vi "prototype UI.vi"() -> ()   [LabVIEW 2012]
uses:
  Custom Controls/Ch selector.ctl
  Custom Controls/MAIN Image panel tab Control type def.ctl
  Custom Controls/scan mode main settings tab.ctl
  Custom Controls/speed mode type def.ctl
  Custom Controls/pixel resolution enum.ctl
  Custom Controls/advanced settings inner tab CTL.ctl
  Custom Controls/Histogram tab.ctl
  Custom Controls/file format type def.ctl
  Custom Controls/experiment type.ctl
  Custom Controls/display palette control.ctl
  Custom Controls/PositionSaveMod.ctl
  <vilib>/event_ctls.llb/lveventtype.ctl
  GFG/GFG library.lvlib
panel:
  in  "PositionSaveButton":T1
  in  "reset zoom":bool
  out "Channel 5 large":T2(plugin-control)
  in  "bool.stage.speed":bool
  in  "Stage Stop":bool
  in  "step.size.xy":u16(ring)=6 items=["  1"=1, "  2"=2, "  5"=5, " 10"=10, " 20"=20, " 50"=50, "100"=100]
  in  "Y UP":bool
  in  "X LEFT":bool
  in  "Y DOWN":bool
  in  "X RIGHT":bool
  out "String 6":string
  in  "shutter":bool
  in  "x.pixels":i32=256 min=2 max=2048 step=2
  in  "clear prot":bool
  in  "timestamp.prot":bool
  in  "protocol.notes":string caption="notebook"
  in  "pos \nstore F":bool
  in  "pos \nstore E":bool
  in  "pos \nstore D":bool
  in  "pos \nstore C":bool
  in  "pos \nstore B":bool
  in  "pos \nstore A":bool
  out "String 10":string
  in  "pos \nrecall F":bool
  in  "pos \nrecall E":bool
  in  "pos \nrecall D":bool
  in  "pos \nrecall C":bool
  in  "pos \nrecall B":bool
  in  "pos \nrecall A":bool
  out "String 11":string
  in  "ref img\nOpen Files Button":bool
  in  "ref img\nstore F":bool
  in  "ref img\nstore E":bool
  in  "ref img\nstore D":bool
  in  "ref img\nstore C":bool
  in  "ref img\nstore B":bool
  in  "ref img\nstore A":bool
  out "String 17":string
  in  "ref img\nSave As Button":bool
  in  "Open All\nSettings":bool
  in  "step.size.z":u16(ring)=6 items=["  1"=1, "  2"=2, "  5"=5, " 10"=10, " 20"=20, " 50"=50, "100"=100]
  out "frame count":dbl(slide) scale=-1.0..280.0
  in  "scan mode main settings":T3
  in  "pixel resolution":T4
  in  "speed mode":T5=2 items=["extra fast scan", "fast scan", "standard scan", "long exposure"]
  in  "ROTATE":dbl(knob)=1.0 min=0.0 max=360.0 step=1.0 scale=0.0..360.0 scale format="%#_3g"
  in  "rotate.enable":bool
  in  "ZOOM":dbl(slide)=1.0 min=1.0 max=10.2 step=0.1 scale=1.0..8.0 scale format="%_2g"
  in  "no. of frames to acquire":i32=10000 min=2 max=2147483646 step=2
  in  "x.fov":dbl caption="Field of view    x" format="%#_3p"
  in  "y.fov":dbl caption="y" format="%#_3p"
  out "ms.p.line":dbl caption="ms/line" format="%#.2g"
  out "frames.p.sec":dbl caption="frames/s" format="%#.2g"
  out "pixels per line":i32=10000 min=2 max=2147483646 step=2
  out "lines per second":i32=10000 min=2 max=2147483646 step=2
  in  "linescan.y.pixels":i32=256 caption="Lines to display at once" min=2 max=2048 step=2
  in  "no. of lines to acquire":i32=10000 min=2 max=2147483646 step=2
  in  "experiment type":T6
  in  "experiment name":string
  in  "root.path":path=path "g:/"
  in  "Objective":u16(ring) items=["40x Olympus", "20x Olympus"]
  in  "file format":T7
  out "stack.duration":i32=10 caption="stack.duration (sec)" min=0 max=2147483646 step=2
  in  "add":bool
  in  "clear all":bool
  in  "clear last":bool
  in  "move to z.stack.\nstart plane":bool
  in  "start z.stack":bool
  in  "frames.per.plane":i32=10000
  in  "z.spacing":dbl=1.0 caption="z.spacing (um)" min=0.1 step=0.1
  out "no of planes":i32=10 min=0 max=2147483646 step=2
  in  "piezo.active":bool
  in  "frames.per.z.cycle":dbl=2.0 min=2.0 max=100.0 step=1.0
  in  "piezo.mode":bool
  in  "Z UP":bool
  in  "Z DOWN":bool
  out "String 7":string
  in  "setY":dbl caption="Z-Stepper" format="%#.1f"
  in  "setX":dbl caption="Z-Stepper" format="%#.1f"
  in  "setZ":dbl caption="set" format="%#.1f"
  out "String 4":string
  out "posZ":dbl caption="actual" format="%#.1f"
  out "posX":dbl caption="Z-Stepper" format="%#.1f"
  out "posY":dbl caption="Z-Stepper" format="%#.1f"
  out "String 3":string
  in  "XYZ stage settings slider tab":enum32{" "}(tab)
  in  "set stage speed":bool
  in  "enable virtual XYZ":bool
  out "String 16":string
  in  "set Y to zero":bool
  in  "set X to zero":bool
  in  "set all to zero":bool
  in  "set Z to zero":bool
  out "String 9":string
  in  "reverse y":bool
  in  "reverse x":bool
  in  "reverse z":bool
  out "String 8":string
  in  "PIN Button XYZ stage settings slider tab":bool
  in  "QUIT":bool
  in  "Record":bool
  in  "FOCUS":bool
  in  "MAIN Image panels":T8
  out "Channel 1 large":T2(plugin-control)
  out "Channel 2 large":T2(plugin-control)
  out "Channel 3 large":T2(plugin-control)
  out "Channel 4 large":T2(plugin-control)
  out "Channel 1 small":T2(plugin-control)
  out "Channel 2 small":T2(plugin-control)
  out "Channel 4 small":T2(plugin-control)
  out "Channel 3 small":T2(plugin-control)
  in  "Blue Channel (Overlay)":T9 caption="B"
  in  "Green Channel (Overlay)":T9=enum."Ch 1" caption="G"
  in  "Red Channel (Overlay)":T9=enum."Ch 2" caption="R"
  out "RGB overlay":T2(plugin-control)
  out "ROI chart":sgl[][](graph)=[[54.570076, 54.556858]]
  in  "ROI channel":T9=enum."Ch 1" caption="Channel"
  out "ROI Image display":T2(plugin-control)
  in  "load coordinates":bool
  in  "confirm line":bool
  in  "channel arb line scan":T9 caption="Channel"
  out "arb line scan display":T2(plugin-control)
  in  "Cancel":bool
  in  "hist/ref slider tab":enum32{" "}(tab)
  in  "PIN Button hist/ref slider tab":bool
  in  "Histograms tab":T10
  in  "auto scale\n      CH 1":bool=TRUE caption="auto scale 2"
  in  "Min Max Channel 1":cluster{dbl, dbl}(slide) scale=-100.0..2047.0 scale format="%#_4g"
  out "Histogram 1":T11(graph)
  out "String 12":string
  in  "auto scale\n      CH 4":bool=TRUE caption="auto scale 2"
  in  "Min Max Channel 4":cluster{dbl, dbl}(slide) scale=-100.0..2047.0 scale format="%#_4g"
  out "Histogram 4":T11(graph)
  out "String 15":string
  in  "auto scale\n      CH 3":bool=TRUE caption="auto scale 2"
  in  "Min Max Channel 3":cluster{dbl, dbl}(slide) scale=-100.0..2047.0 scale format="%#_4g"
  out "Histogram 3":T11(graph)
  out "String 14":string
  in  "auto scale\n      CH 2":bool=TRUE caption="auto scale 2"
  in  "Min Max Channel 2":cluster{dbl, dbl}(slide) scale=-100.0..2047.0 scale format="%#_4g"
  out "Histogram 2":T11(graph)
  out "String 13":string
  in  "avg type":u16(ring) items=["none", "group avg", "moving avg"]
  in  "avg of":i8=10 min=2 step=1
  in  "display palette":T12
  in  "laser power slider tab":enum32{""}(tab)
  in  "enable set power max":bool
  in  "set power max":bool
  in  "Laser Power":dbl(knob) step=0.5 scale=0.0..100.0 scale format="%3d"
  in  "PIN Button laser power slider tab":bool
  in  "PMT slider tab":enum32{""}(tab)
  in  "PMT 2":u16(slide) max=1000 scale=0.0..1000.0
  in  "PMT 1":u16(slide) max=1250 scale=0.0..1000.0
  out "String 5":string
  in  "PMT 4":u16(slide) max=1000 scale=0.0..1000.0
  in  "PMT 3":u16(slide) max=1250 scale=0.0..1000.0
  out "String 18":string
  in  "PIN Button PMT slider tab":bool
  in  "advanced settings slider tab":enum32{""}(tab)
  in  "advanced settings inner tab":T13
  in  "pixel.dwell.time.in.sec":dbl=1e-05 min=4e-07 max=1e-05 step=2e-07 format="%#.6p"
  in  "y.pixel.sz":dbl=1e-05 min=1e-09 max=1e-05 step=1e-07 format="%#_3p"
  in  "x.pixel.sz":dbl=1e-05 min=1e-09 max=1e-05 step=1e-07 format="%#_3p"
  in  "y.pixels":i32=256 caption="Y Resolution" min=2 max=2048 step=2
  in  "fill fraction":dbl=60.0 caption="%" min=60.0 max=100.0 step=0.5 format="%_3g"
  in  "nomin.x.pixels":i32=256 caption="X resolution" min=2 max=2048 step=2
  in  "y bidirectional":bool
  in  "x bidirectional":bool=TRUE
  in  "max.field.of.view":dbl=300.0 format="%#_6p"
  in  "voltage.for\nmax.field.of.view":dbl=5.0
  in  "x.voltage":dbl=0.9999999999999999 min=0.0 max=5.5 step=0.1
  in  "y.voltage":dbl=1.0 min=0.0 max=5.5 step=0.1
  in  "y.volt.offset":dbl=-0.2 step=0.1
  in  "x.volt.offset":dbl=-0.2 step=0.1
  in  "pixel.dwell.time.in.ticks":u16=20 min=2 step=1
  in  "sample.clock":dbl=5000000.0
  in  "Start.Delay":dbl=100.0 min=1.0 step=1.0
  out "ADsamples.per.frame":i32
  in  "ai.active3":bool
  in  "ai.active2":bool
  in  "ai.active1":bool
  in  "ai.active0":bool caption="active?"
  in  "ai.range2":dbl=10.0 min=0.1 max=10.0 step=0.1
  in  "ai.range1":dbl=10.0 min=0.1 max=10.0 step=0.1
  out "ai.string3":string
  out "ai.string2":string
  out "ai.string1":string
  out "ai.string0":string caption="Analog Input"
  in  "ai.range0":dbl=10.0 caption="input range" min=0.1 max=10.0 step=0.1
  in  "ai.range3":dbl=10.0 min=0.1 max=10.0 step=0.1
  in  "external.start.trigger.enable":bool=TRUE caption="WAIT FOR TRIGGER"
  in  "pos  pockels cell PMT Data":dbl[][](array[numeric])=[[0.0, 0.0], [1.0, 0.0]] caption="Data" format="%0.1f"
  out "interpol XY":cluster{dbl[], "Best Exponential Fit":dbl[]}[](graph)
  in  "PIN Button advanced settings slider tab":bool
  in  "SCIENTIFICA Button":bool
  # "to zoom out press and hold Shift"
  # "current pos."
  # "go to pos."
  # "STORE positions"
  # "RECALL  positions"
  # "REFERENCE IMAGES"
  # "STORE"
  # "zig-zag (leaf scan)"
  # "planes"
  # "virtual XYZ"
  # "set zero"
  # "reverse \ndirection"
  # "1"
  # "2"
  # "3"
  # "4"
  # "Press and hold Ctrl to add multriple ROIs"
  # "This checkbox is only for starting the image acquisition using a TTL rising edge trigger from an external device. Don't tick this box unless an incoming trigger is wired up, otherwise the software may freeze. To reset, click QUIT and restart. If you want to send a trigger to an external device, just connect the ai.start.trigger.channel (e.g.PFI2, specified in settings.INI) to the external device, but leave the  checkbox above unticked."
  # "Z"
  # "laser"
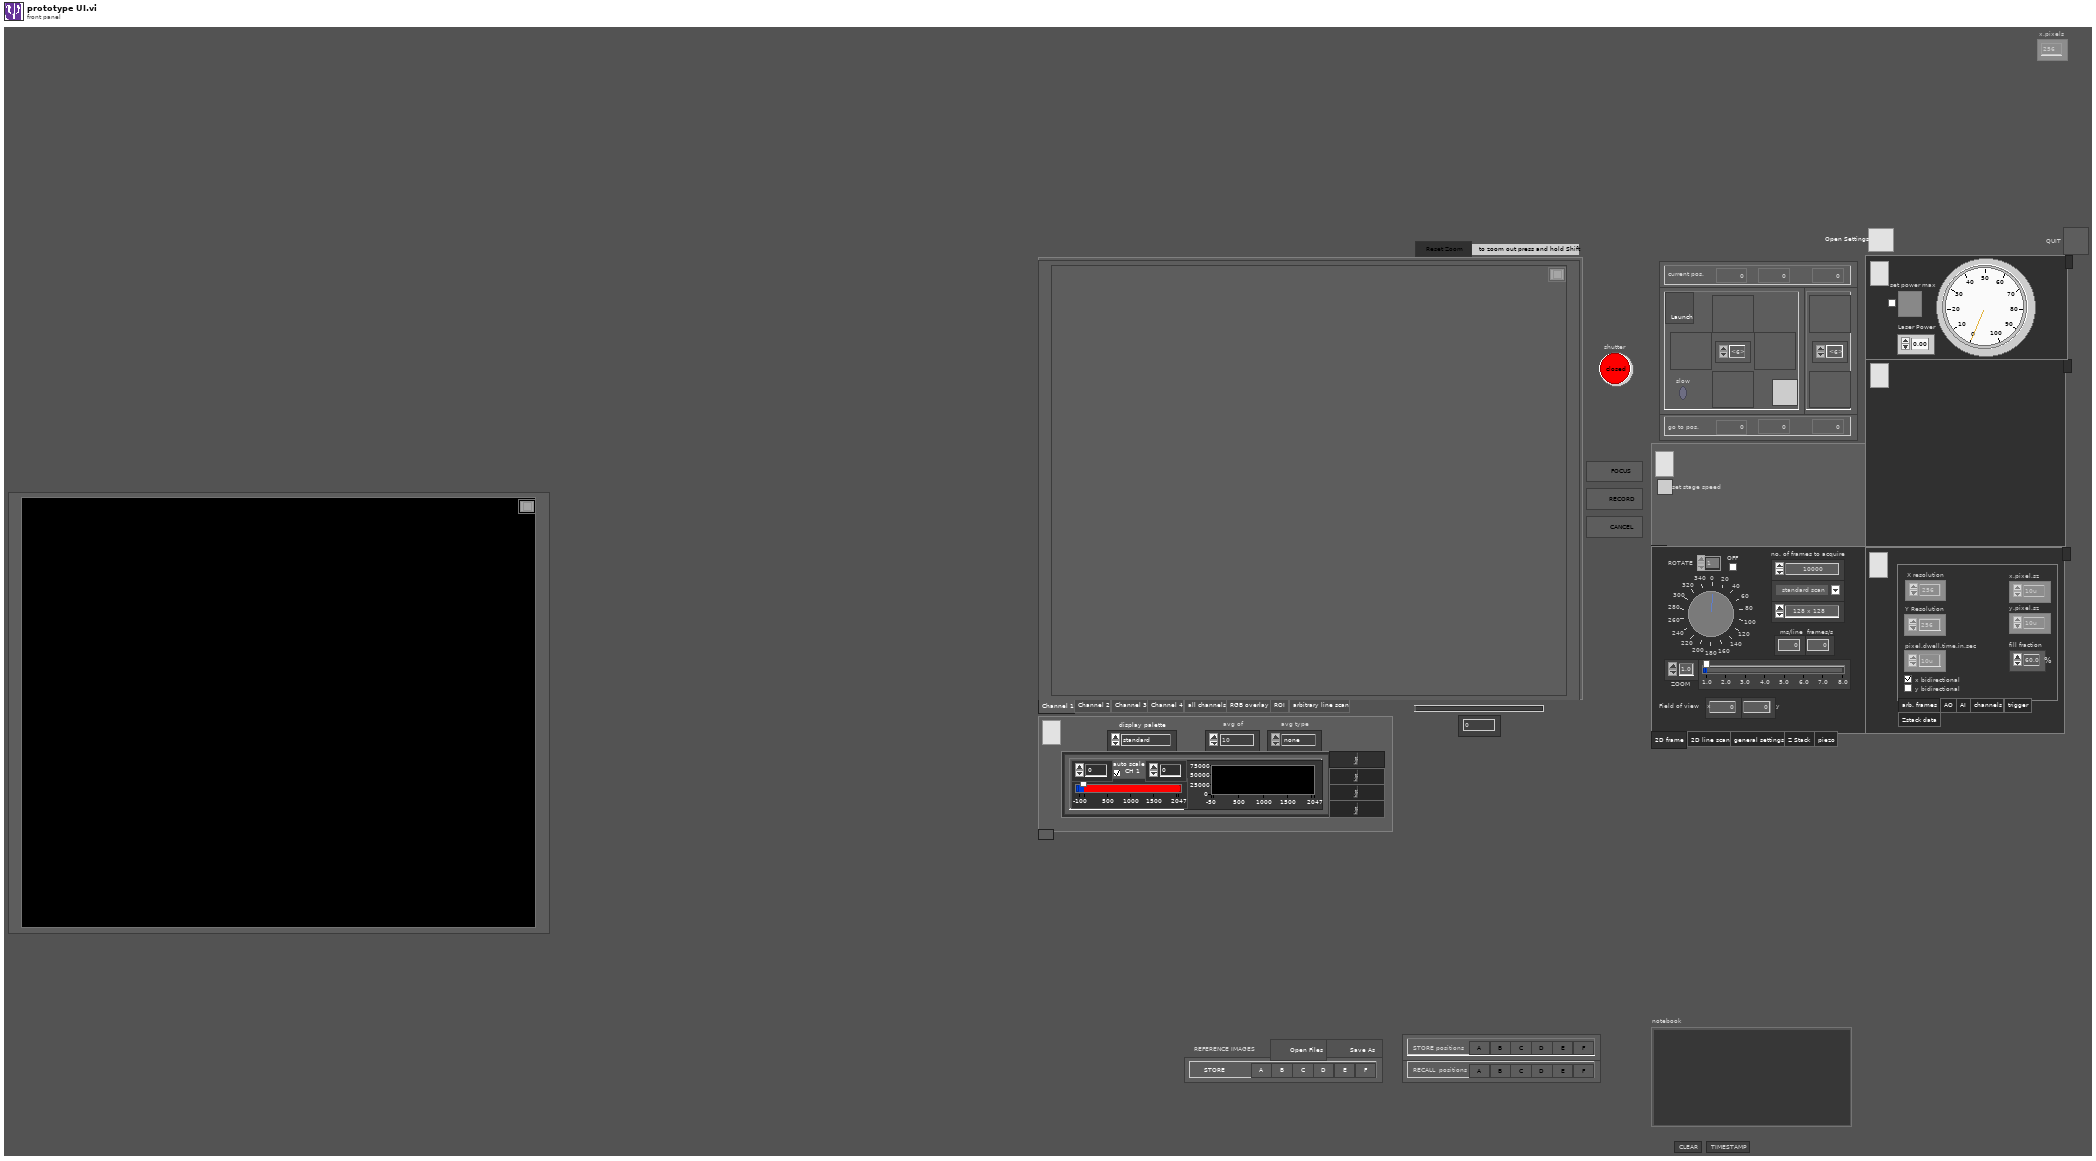
[diagram p1: front panel]
types:
  T1 = typedef "PositionSaveMod.ctl" = bool
  T2 = typedef "IMAQ Image.ctl" = refnum<image>
  T3 = typedef "scan mode main settings tab.ctl" = enum32{"2D frame", "2D line scan", "general settings", "Z Stack", "piezo"}
  T4 = typedef "pixel resolution enum.ctl" = enum16{"   128 x 128", "   256 x 128", "   256 x 256", "   512 x  64", "   512 x 128", "   512 x 256", "   512 x 512", "  1024 x 512", "  1024 x 1024", "   arbitrary"}
  T5 = typedef "speed mode type def.ctl" = u16
  T6 = typedef "experiment type.ctl" = string
  T7 = typedef "file format type def.ctl" = enum16{"16bit raw", "32bit raw", "16bit multi-tiff (interleave)", "16bit multi-tiff (separate)", "16bit multi-tiff (stacked)", "32bit multi-tiff (interleave)", "32bit multi-tiff (separate)", "32bit multi-tiff (stacked)", "16bit tiff series (interleave)", "16bit tiff series (separate)", "16bit tiff series (stacked)", "32bit tiff series (interleave)", "32bit tiff series (separate)", "32bit tiff series (stacked)"}
  T8 = typedef "MAIN Image panel tab Control type def.ctl" = enum32{"Channel 1", "Channel 2", "Channel 3", "Channel 4", "all channels", "RGB overlay", "ROI", "arbitrary line scan"}
  T9 = typedef "Ch selector.ctl" = enum16{"none", "Ch 1", "Ch 2", "Ch 3", "Ch 4", "Ch 5"}
  T10 = typedef "Histogram tab.ctl" = enum32{"hist Ch 1", "hist Ch 4", "hist Ch 3", "hist Ch 2"}
  T11 = cluster{"Starting Value":sgl, "Incremental Value":sgl, "Histogram":u32[]}
  T12 = typedef "display palette control.ctl" = enum16{"standard", "high clipping red", "low clipping blue", "high and low clipping"}
  T13 = typedef "advanced settings inner tab CTL.ctl" = enum32{"arb. frames", "AO", "AI", "channels", "trigger", "Zstack data"}
  T14 = enum8{"Enabled", "Disabled", "Disabled and Grayed Out"}
  T15 = typedef "Image Type" = u32
  T16 = cluster{refnum<vi>, refnum<vi>, refnum<vi>, refnum<vi>, refnum<vi>, refnum<vi>, refnum<vi>, refnum<vi>, refnum<vi>, refnum<vi>, refnum<vi>, refnum<vi>}
  T17 = cluster{"New Image":T2, "New Image":T2, "New Image":T2, "New Image":T2, "New Image":T2, "New Image":T2, "New Image":T2, "New Image":T2, "New Image":T2, "New Image":T2, "New Image":T2, "New Image":T2}
  T18 = typedef "lveventtype.ctl" = enum32{"Null", "Timeout", "Annotation Menu Selection", "Annotation Menu Selection?", "App Instance Close", "App Instance Close?", "Autoscale Range Change", "Cell Edit", "Cell Edit?", "Cursor Grab", "Cursor Grab?", "Cursor Menu Selection", "Cursor Menu Selection?", "Cursor Move", "Cursor Release", "Data Change", "Direction Change", "Display State Change", "Drag Ended", "Drag Enter", "Drag Leave", "Drag Over", "Drag Source Update", "Drag Starting", "Drag Starting?", "Drop", "Exec State Change", "Key Down", "Key Down?", "Key Repeat", "Key Repeat?", "Key Up", "Listbox Double Click", "Menu Activation?", "Menu Selection (App)", "Menu Selection? (App)", "Menu Selection (User)", "Mouse Down", "Mouse Down?", "Mouse Enter", "Mouse Leave", "Mouse Move", "Mouse Up", "NI Security User Change (App)", "Pane Size", "Panel Close", "Panel Close?", "Panel Resize", "Plot Attribute Change", "Scale Range Change", "Shortcut Menu Activation?", "Shortcut Menu Selection (App)", "Shortcut Menu Selection? (App)", "Shortcut Menu Selection (User)", "Tree Double Click", "Tree Drag", "Tree Drag?", "Tree Drop", "Tree Drop?", "Tree Item Close", "Tree Item Close?", "Tree Item Open", "Tree Item Open?", "Value Change"}
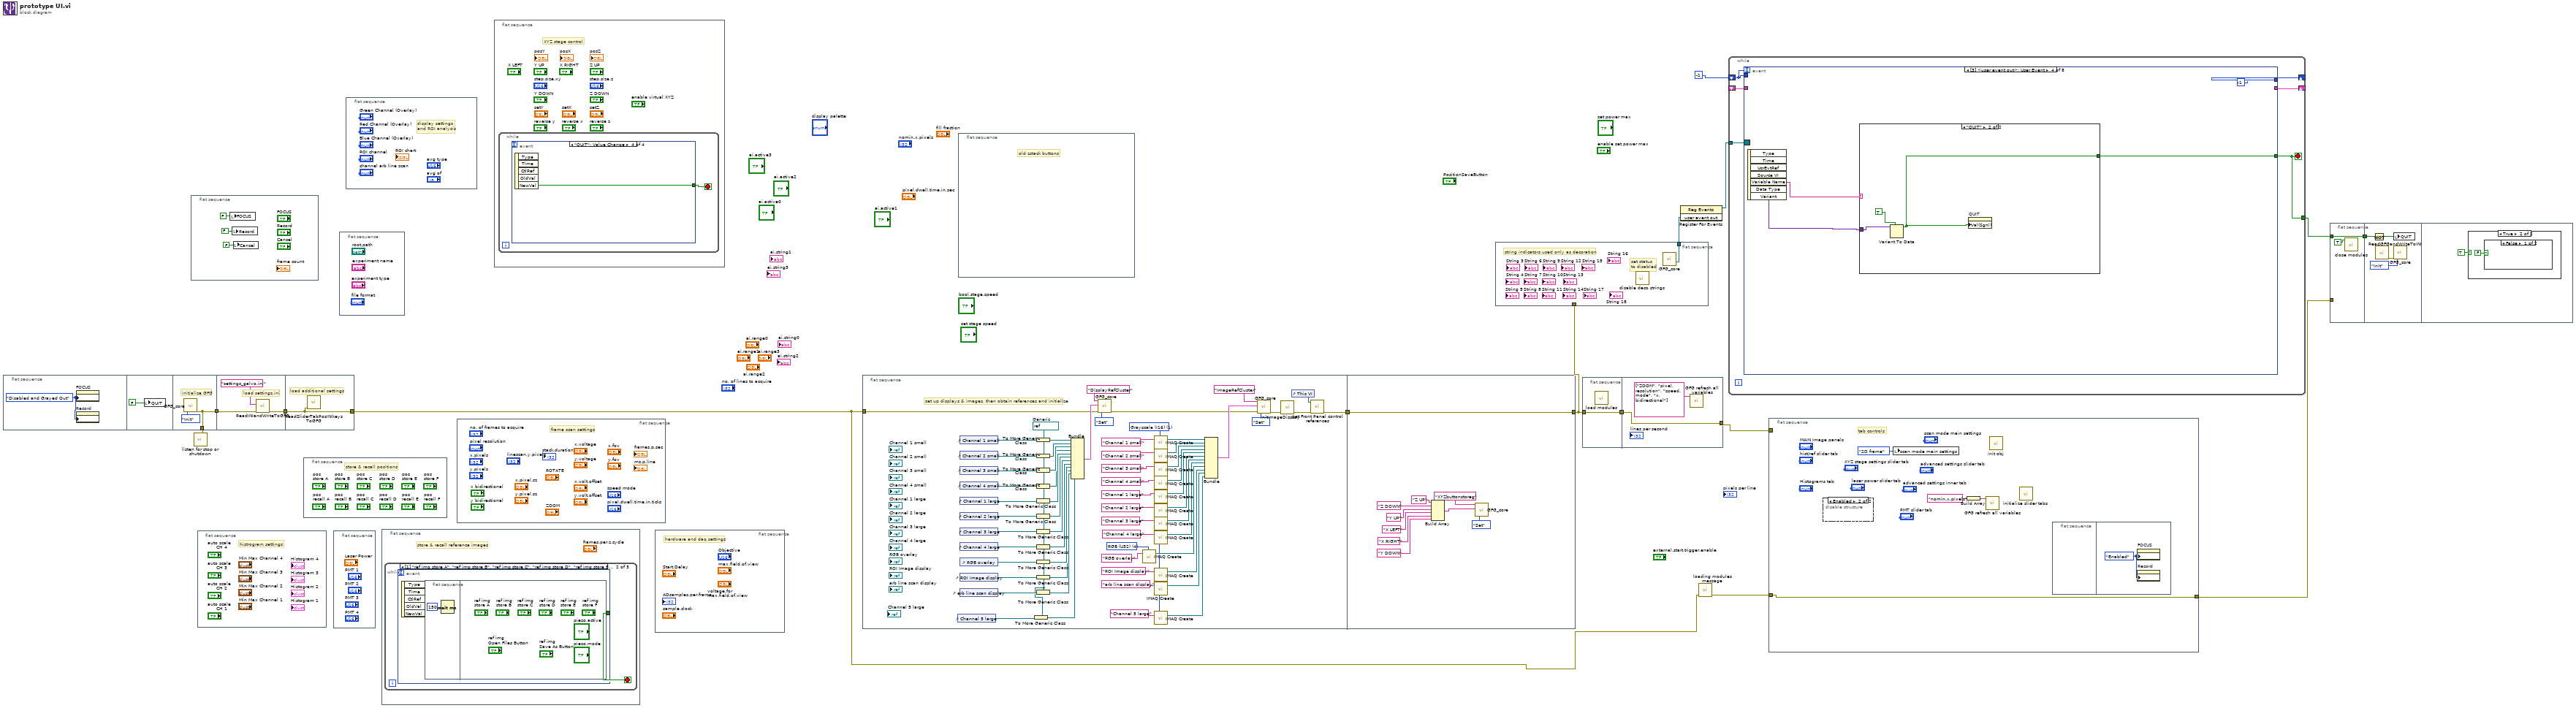
[diagram p0: block diagram]
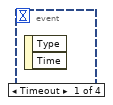
[diagram p2: hidden frame]
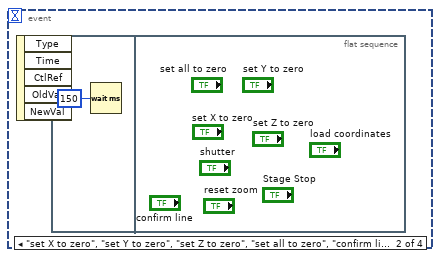
[diagram p3: hidden frame]
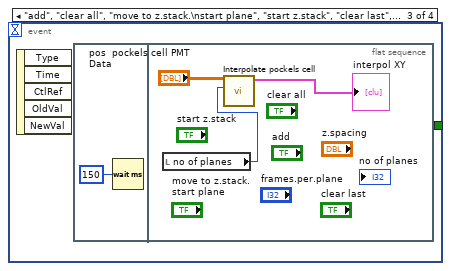
[diagram p4: hidden frame]
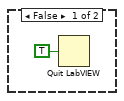
[diagram p5: hidden frame]
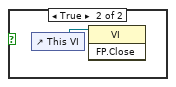
[diagram p6: hidden frame]
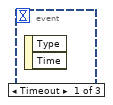
[diagram p7: hidden frame]
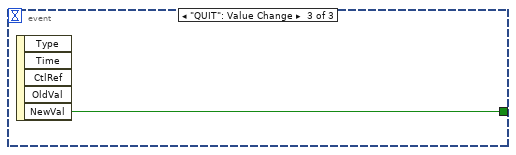
[diagram p8: hidden frame]
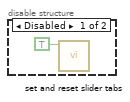
[diagram p9: hidden frame]
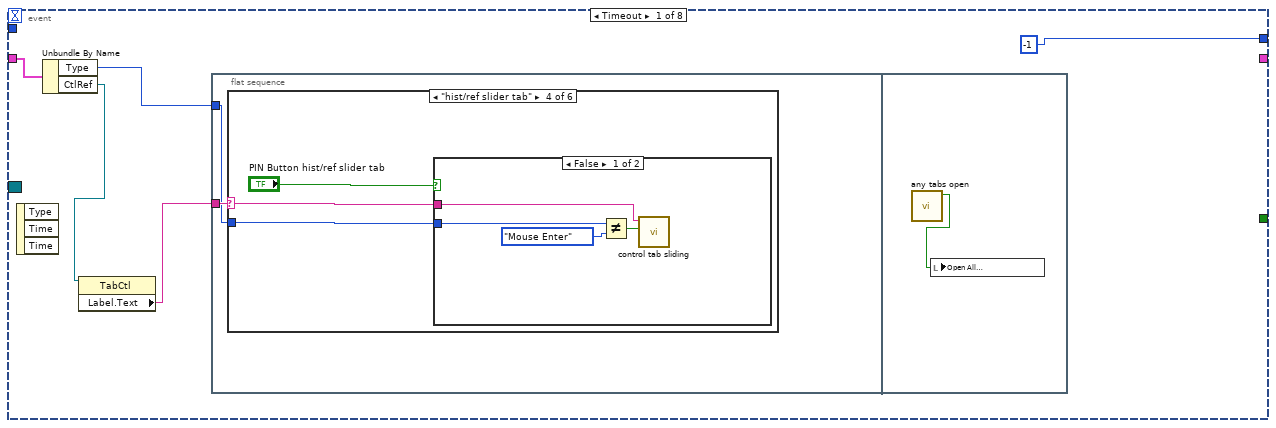
[diagram p10: hidden frame]
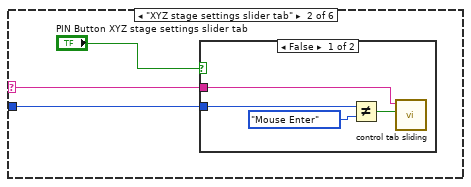
[diagram p12: hidden frame]
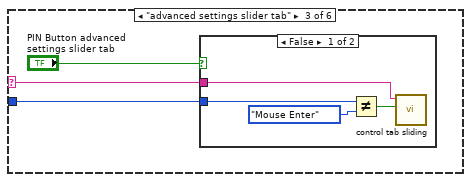
[diagram p14: hidden frame]
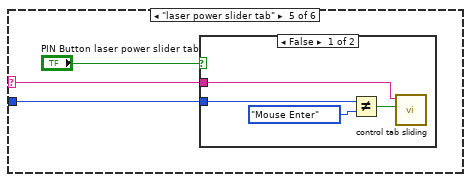
[diagram p17: hidden frame]
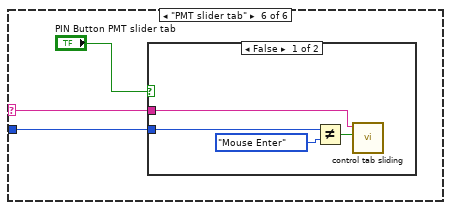
[diagram p19: hidden frame]
diagram:
  n1 = flat-sequence {
    tunnel: [w18] -> w15
    tunnel: [w18] -> w14
    tunnel: w15 -> [w22]
    tunnel: [w21] -> w9
    tunnel: [w23] -> w4
    tunnel: w9 -> [w23]
    frame #0 {
      w16 = T14."Disabled and Grayed Out" ("Disabled")
      n2 = property on="FOCUS" class="Bool (strict)"("DisabledEnum"=w16) -> ()  [unwired: 2 in, 2 out]
      n3 = property on="Record" class="Bool (strict)"("DisabledEnum"=w16) -> ()  [unwired: 2 in, 2 out]
    }
    frame #1 {
      n4 = local write "QUIT"(FALSE ("QUIT")) -> ()
    }
    frame #2 {
      # "initialize GFG"
      n5 = call "GFG_core.vi"("Action"=enum16{"Init", "Set", "Get"}."Init") -> ("error out"=w18:errorcluster)  [unwired: 12 in, 6 out]
    }
    frame #3 {
      # "load settings.ini"
      n6 = call "ReadINIandWriteToGFG.vi"("error in (no error)"=w22, "name or relative path"="settings_galvo.ini") -> ("error out"=w21:errorcluster)  [unwired: 9 in]
    }
    frame #4 {
      # "load additional settings"
      n7 = call "ReadSliderTabPosINIkeysToGFG.vi"("error in (no error)"=w23) -> ()  [unwired: 11 in]
    }
  }
  n8 = flat-sequence {
    frame #0 {
      n9 = local write "FOCUS"(FALSE ("FOCUS")) -> ()
      n10 = local write "Record"(FALSE ("Record")) -> ()
      n11 = local write "Cancel"(FALSE ("Cancel")) -> ()
    }
  }
  n12 = call "listen for stop or shutdown.vi"("error in (no error)"=w14) -> ()  [unwired: 9 in, 2 out]
  n13 = flat-sequence {
    frame #0 {
      # "histrogram settings"
    }
  }
  n14 = flat-sequence {
    frame #0 {
      # "store & recall positions"
    }
  }
  n15 = flat-sequence {
    frame #0 {
    }
  }
  n16 = flat-sequence {
    frame #0 {
    }
  }
  n17 = flat-sequence {
    frame #0 {
      # "display settings\nand ROI analysis"
    }
  }
  n18 = flat-sequence {
    frame #0 {
      # "store & recall reference images"
      n19 = while {
        stop <- w27 stop-if-true
        n20 = event shown="[1] \"ref img store A\", \"ref img store B\", \"ref img store C\", \"ref img store D\", \"ref img store E\", \"ref img store F\", \"ref img Save As Button\", \"ref img Open Files Button\": Value Change" {
          selector: _ -> [_ _ _]
          dyn-events: _ -> [_ _ _]
          timeout: _ -> [_ _ _]
          tunnel: [_ _ w29] -> w27
          event Timeout {
            n21 = event-data() -> ()  [unwired: 1 in, 2 out]
          }
          event "ref img\nstore A", "ref img\nstore B", "ref img\nstore C", "ref img\nstore D", "ref img\nstore E", "ref img\nstore F", "ref img\nSave As Button", "ref img\nOpen Files Button": Value Change {
            n22 = event-data() -> ()  [unwired: 1 in, 5 out]
            n23 = flat-sequence {
              frame #0 {
                n24 = Wait (ms)(milliseconds to wait=u32 150) -> ()  [unwired: 1 out]
              }
              frame #1 {
              }
            }
          }
          event "QUIT": Value Change {
            n25 = event-data() -> ("NewVal"=w29:bool)  [unwired: 1 in, 4 out]
          }
        }
      }
    }
  }
  n26 = flat-sequence {
    frame #0 {
      # "frame scan settings"
    }
  }
  n27 = flat-sequence {
    frame #0 {
      # "XYZ stage control"
      n28 = while {
        stop <- w30 stop-if-true
        n29 = event shown="[3] \"QUIT\": Value Change" {
          selector: _ -> [_ _ _ _]
          dyn-events: _ -> [_ _ _ _]
          timeout: _ -> [_ _ _ _]
          tunnel: [_ _ _ w36] -> w30
          event Timeout {
            n30 = event-data() -> ()  [unwired: 1 in, 2 out]
          }
          event "set X to zero", "set Y to zero", "set Z to zero", "set all to zero", "confirm line", "Stage Stop", "reset zoom": Value Change {
            n31 = event-data() -> ()  [unwired: 1 in, 5 out]
            n32 = flat-sequence {
              frame #0 {
                n33 = Wait (ms)(milliseconds to wait=u32 150) -> ()  [unwired: 1 out]
              }
              frame #1 {
              }
            }
          }
          event "add", "clear all", "move to z.stack.\nstart plane", "start z.stack", "clear last", "z.spacing", "frames.per.plane", "no of planes", "pos  pockels cell PMT Data": Value Change {
            n34 = event-data() -> ()  [unwired: 1 in, 5 out]
            n35 = flat-sequence {
              frame #0 {
                n36 = Wait (ms)(milliseconds to wait=u32 150) -> ()  [unwired: 1 out]
              }
              frame #1 {
                n37 = local read "no of planes"() -> (w33:i32)
                n38 = call "Interpolate pockels cell.vi"("nr of planes"=w33, "Data"="pos  pockels cell PMT Data") -> ("Raw Data and Interpolated Data"=→"interpol XY":cluster{dbl[], "Best Exponential Fit":dbl[]}[])  [unwired: 8 in, 1 out]
              }
            }
          }
          event "QUIT": Value Change {
            n39 = event-data() -> ("NewVal"=w36:bool)  [unwired: 1 in, 4 out]
          }
        }
      }
    }
  }
  n40 = flat-sequence {
    frame #0 {
      # "hardware and daq settings"
    }
  }
  n41 = flat-sequence {
    tunnel: w4 -> [w56]
    tunnel: [w37] -> w6
    tunnel: [w109] -> w12
    tunnel: w6 -> [w109]
    frame #0 {
      w44 = T15 4 items=["Grayscale (U8)", "Grayscale (I16)", "Grayscale (SGL)", "Complex (CSG)", "RGB (U32)", "HSL (U32)", "RGB (U64)", "Grayscale (U16)"] ("Image Type")
      w39 = T15 1 items=["Grayscale (U8)", "Grayscale (I16)", "Grayscale (SGL)", "Complex (CSG)", "RGB (U32)", "HSL (U32)", "RGB (U64)", "Grayscale (U16)"] ("Image Type")
      w41 = refnum<vi> refnum  # Generic
      # "set up displays & images, then obtain references and initialize"
      n42 = control-ref of="Channel 5 large"() -> (w43:refnum<vi>)
      n43 = control-ref of="Channel 1 small"() -> (w55:refnum<vi>)
      n44 = control-ref of="Channel 2 small"() -> (w54:refnum<vi>)
      n45 = control-ref of="Channel 3 small"() -> (w53:refnum<vi>)
      n46 = control-ref of="Channel 4 small"() -> (w52:refnum<vi>)
      n47 = control-ref of="Channel 1 large"() -> (w51:refnum<vi>)
      n48 = control-ref of="Channel 2 large"() -> (w50:refnum<vi>)
      n49 = control-ref of="Channel 3 large"() -> (w49:refnum<vi>)
      n50 = control-ref of="Channel 4 large"() -> (w48:refnum<vi>)
      n51 = control-ref of="RGB overlay"() -> (w47:refnum<vi>)
      n52 = control-ref of="ROI Image display"() -> (w46:refnum<vi>)
      n53 = control-ref of="arb line scan display"() -> (w45:refnum<vi>)
      n54 = To More Generic Class(target class=w41, reference=w43) -> (generic class reference=w40:refnum<vi>)
      n55 = To More Generic Class(target class=w41, reference=w55) -> (generic class reference=w96:refnum<vi>)
      n56 = To More Generic Class(target class=w41, reference=w54) -> (generic class reference=w89:refnum<vi>)
      n57 = To More Generic Class(target class=w41, reference=w53) -> (generic class reference=w88:refnum<vi>)
      n58 = To More Generic Class(target class=w41, reference=w52) -> (generic class reference=w87:refnum<vi>)
      n59 = To More Generic Class(target class=w41, reference=w51) -> (generic class reference=w86:refnum<vi>)
      n60 = To More Generic Class(target class=w41, reference=w50) -> (generic class reference=w95:refnum<vi>)
      n61 = To More Generic Class(target class=w41, reference=w49) -> (generic class reference=w94:refnum<vi>)
      n62 = To More Generic Class(target class=w41, reference=w48) -> (generic class reference=w93:refnum<vi>)
      n63 = To More Generic Class(target class=w41, reference=w47) -> (generic class reference=w92:refnum<vi>)
      n64 = To More Generic Class(target class=w41, reference=w46) -> (generic class reference=w91:refnum<vi>)
      n65 = To More Generic Class(target class=w41, reference=w45) -> (generic class reference=w90:refnum<vi>)
      n66 = Bundle(w96, w89, w88, w87, w86, w95, w94, w93, w92, w91, w90, w40) -> (w99:T16)  [unwired: 1 in]
      n67 = call "GFG_core.vi"("Variable Name in"="DisplayRefCluster", "Variant in"=w99, "error in (no error)"=w56, "Action"=enum16{"Init", "Set", "Get"}."Set") -> ("error out"=w60:errorcluster)  [unwired: 9 in, 6 out]
      n68 = call "IMAQ Create"("Image Name"="RGB overlay", "Image Type"=w44) -> ("New Image"=w80:T2)  [unwired: 3 in, 1 out]
      n69 = call "IMAQ Create"("Image Name"="Channel 1 small", "Image Type"=w39) -> ("New Image"=w72:T2)  [unwired: 3 in, 1 out]
      n70 = call "IMAQ Create"("Image Name"="Channel 2 small", "Image Type"=w39) -> ("New Image"=w73:T2)  [unwired: 3 in, 1 out]
      n71 = call "IMAQ Create"("Image Name"="Channel 3 small", "Image Type"=w39) -> ("New Image"=w74:T2)  [unwired: 3 in, 1 out]
      n72 = call "IMAQ Create"("Image Name"="Channel 4 small", "Image Type"=w39) -> ("New Image"=w75:T2)  [unwired: 3 in, 1 out]
      n73 = call "IMAQ Create"("Image Name"="Channel 1 large", "Image Type"=w39) -> ("New Image"=w76:T2)  [unwired: 3 in, 1 out]
      n74 = call "IMAQ Create"("Image Name"="Channel 2 large", "Image Type"=w39) -> ("New Image"=w77:T2)  [unwired: 3 in, 1 out]
      n75 = call "IMAQ Create"("Image Name"="Channel 3 large", "Image Type"=w39) -> ("New Image"=w78:T2)  [unwired: 3 in, 1 out]
      n76 = call "IMAQ Create"("Image Name"="Channel 4 large", "Image Type"=w39) -> ("New Image"=w79:T2)  [unwired: 3 in, 1 out]
      n77 = call "IMAQ Create"("Image Name"="ROI Image display", "Image Type"=w39) -> ("New Image"=w81:T2)  [unwired: 3 in, 1 out]
      n78 = call "IMAQ Create"("Image Name"="arb line scan display", "Image Type"=w39) -> ("New Image"=w82:T2)  [unwired: 3 in, 1 out]
      n79 = call "IMAQ Create"("Image Name"="Channel 5 large", "Image Type"=w39) -> ("New Image"=w38:T2)  [unwired: 3 in, 1 out]
      n80 = Bundle("New Image"=w72, "New Image"=w73, "New Image"=w74, "New Image"=w75, "New Image"=w76, "New Image"=w77, "New Image"=w78, "New Image"=w79, "New Image"=w80, "New Image"=w81, "New Image"=w82, "New Image"=w38) -> (w84:T17)  [unwired: 1 in]
      n81 = call "GFG_core.vi"("Variable Name in"="ImageRefCluster", "Variant in"=w84, "error in (no error)"=w60, "Action"=enum16{"Init", "Set", "Get"}."Set") -> ("error out"=w59:errorcluster)  [unwired: 9 in, 6 out]
      n82 = call "InitImageDisplay.vi"("error in (no error)"=w59) -> ("error out"=w58:errorcluster)  [unwired: 10 in]
      n83 = control-ref of="This VI"() -> (w57:refnum<vi>)
      n84 = call "get Front Panel control references.vi"("error in (no error)"=w58, "Main VI"=w57) -> ("error out"=w37:errorcluster)  [unwired: 9 in]
    }
    frame #1 {
      n85 = Build Array("Z UP" ("Variable Name in"), "Z DOWN" ("Variable Name in"), "Y UP" ("Variable Name in"), "X LEFT" ("Variable Name in"), "X RIGHT" ("Variable Name in"), "Y DOWN" ("Variable Name in")) -> (w100:string[])
      n86 = call "GFG_core.vi"("Variable Name in"="XYZbuttonstoreg", "Variant in"=w100, "Action"=enum16{"Init", "Set", "Get"}."Set") -> ()  [unwired: 10 in, 7 out]
    }
  }
  n87 = flat-sequence {
    frame #0 {
      # "old zstack buttons"
    }
  }
  n88 = flat-sequence {
    tunnel: w12 -> [_]
    tunnel: [w110] -> w2
    frame #0 {
      # "set status\nto disabled"
      # "string indicators used only as decoration"
      n89 = call "disable deco strings.vi"() -> ()  [unwired: 11 in, 1 out]
      n90 = call "GFG_core.vi"() -> ("user event out"=w110:refnum<user-event>)  [unwired: 13 in, 6 out]
    }
  }
  n91 = flat-sequence {
    tunnel: w12 -> [w111]
    tunnel: [w111] -> w8
    tunnel: [w113] -> w7
    tunnel: w8 -> [w113]
    frame #0 {
      n92 = call "load modules.vi"() -> ()  [unwired: 12 in]
    }
    frame #1 {
      n93 = call "GFG refresh all variables.vi"("Variables to refresh"=string[] ["ZOOM", "pixel.resolution", "speed.mode", "x.bidirectional"] ("Variables Names In")) -> ()  [unwired: 11 in]
    }
  }
  n94 = register-events(w2) -> (reference out=w3:refnum<event-registration>)  [unwired: 2 in, 1 out]
  n95 = call "loading modules message.vi"("error in"=w4) -> ("error out"=w5:errorcluster)  [unwired: 10 in]
  n96 = while {
    tunnel: [w119] -> w13
    shift-right: [w118] -> _
    shift-left: _ -> [w116]
    shift-right: [w117] -> _
    shift-left: -1 -> [w115]
    tunnel: w3 -> [w114]
    stop <- w119 stop-if-true
    n97 = event shown="[3] <user event out>: User Event" {
      selector: w114 -> [_ _ _ _ _ _ _ _]
      dyn-events: _ -> [_ _ _ _ _ _ _ _]
      timeout: w115 -> [_ _ _ _ _ _ _ _]
      tunnel: [_ _ "QUIT" w177 _ _ _ _] -> w119
      tunnel: [_ _ _ _ _ _ w191 _] -> w118
      tunnel: [-1 w163 w174 -1 w183 w185 w195 w205] -> w117
      tunnel: w116 -> [w124 _ _ _ _ _ w190 _]
      tunnel: w115 -> [_ w163 w174 _ w183 w185 w194 w205]
      event Timeout {
        n98 = event-data() -> ()  [unwired: 1 in, 3 out]
        n99 = Unbundle By Name(w124) -> ("Type"=w121:T18, "CtlRef"=w123:refnum<vi>)
        n100 = property class="TabCtl"(reference=w123) -> ("Label.Text"=w122:string)  [unwired: 1 in, 2 out]
        n101 = flat-sequence {
          tunnel: w122 -> [w126]
          tunnel: w121 -> [w125]
          frame #0 {
            n102 = case shown="\"hist/ref slider tab\"" w126 {
              selector: w126 -> [_ w128 w134 w143 w148 w157]
              tunnel: w125 -> [_ w127 w135 w141 w149 w156]
              frame "False", Default {
              }
              frame "XYZ stage settings slider tab" {
                n103 = case shown="False" "PIN Button XYZ stage settings slider tab" {
                  tunnel: w128 -> [w133 _]
                  tunnel: w127 -> [w132 _]
                  frame False {
                    n104 = Not Equal?(x=w132, y=lveventtype."Mouse Enter" ("Type")) -> (x != y?=w131:bool)
                    n105 = call "control tab sliding.vi"("close(T)/open(F)"=w131, "String"=w133) -> ()  [unwired: 10 in]
                  }
                  frame True {
                  }
                }
              }
              frame "advanced settings slider tab" {
                n106 = case shown="False" "PIN Button advanced settings slider tab" {
                  tunnel: w134 -> [w140 _]
                  tunnel: w135 -> [w139 _]
                  frame False {
                    n107 = Not Equal?(x=w139, y=lveventtype."Mouse Enter" ("Type")) -> (x != y?=w138:bool)
                    n108 = call "control tab sliding.vi"("close(T)/open(F)"=w138, "String"=w140) -> ()  [unwired: 10 in]
                  }
                  frame True {
                  }
                }
              }
              frame "hist/ref slider tab" {
                n109 = case shown="False" "PIN Button hist/ref slider tab" {
                  tunnel: w143 -> [w147 _]
                  tunnel: w141 -> [w146 _]
                  frame False {
                    n110 = Not Equal?(x=w146, y=lveventtype."Mouse Enter" ("Type")) -> (x != y?=w145:bool)
                    n111 = call "control tab sliding.vi"("close(T)/open(F)"=w145, "String"=w147) -> ()  [unwired: 10 in]
                  }
                  frame True {
                  }
                }
              }
              frame "laser power slider tab" {
                n112 = case shown="False" "PIN Button laser power slider tab" {
                  tunnel: w148 -> [w154 _]
                  tunnel: w149 -> [w153 _]
                  frame False {
                    n113 = Not Equal?(x=w153, y=lveventtype."Mouse Enter" ("Type")) -> (x != y?=w152:bool)
                    n114 = call "control tab sliding.vi"("close(T)/open(F)"=w152, "String"=w154) -> ()  [unwired: 10 in]
                  }
                  frame True {
                  }
                }
              }
              frame "PMT slider tab" {
                n115 = case shown="False" "PIN Button PMT slider tab" {
                  tunnel: w157 -> [w161 _]
                  tunnel: w156 -> [w160 _]
                  frame False {
                    n116 = Not Equal?(x=w160, y=lveventtype."Mouse Enter" ("Type")) -> (x != y?=w159:bool)
                    n117 = call "control tab sliding.vi"("close(T)/open(F)"=w159, "String"=w161) -> ()  [unwired: 10 in]
                  }
                  frame True {
                  }
                }
              }
            }
          }
          frame #1 {
            n118 = call "any tabs open.vi"() -> ("any tabs open?"=w162:bool)  [unwired: 11 in]
            n119 = local write "Open All\nSettings"(w162) -> ()
          }
        }
      }
      event "Open All\nSettings": Value Change {
        n120 = event-data() -> ()  [unwired: 1 in, 5 out]
        n121 = case shown="True" "Open All\nSettings" {
          frame False {
            n122 = call "slider tabs open.vi"("close(T)/open(F)"=TRUE) -> ()  [unwired: 11 in]
          }
          frame True {
            n123 = call "slider tabs open.vi"("close(T)/open(F)"=FALSE) -> ()  [unwired: 11 in]
          }
        }
      }
      event "QUIT": Value Change {
        n124 = event-data() -> ()  [unwired: 1 in, 5 out]
        n125 = call "getVIname.vi"() -> ("VI name"=w173:string)  [unwired: 19 in]
        n126 = call "SendShutdownCommand.vi"("Source VI"=w173) -> ()  [unwired: 11 in]
        n127 = call "GFG_core.vi"("Variable Name in"="shutter", "Variant in"=FALSE ("QUIT"), "Action"=enum16{"Init", "Set", "Get"}."Set") -> ()  [unwired: 10 in, 7 out]
        n128 = call "GFG_core.vi"("Variable Name in"="Cancel", "Variant in"=FALSE ("QUIT"), "Action"=enum16{"Init", "Set", "Get"}."Set") -> ()  [unwired: 10 in, 7 out]
      }
      event User Event {
        n129 = event-data() -> ("Variable Name"=w179:string, "Variant"=w178:variant)  [unwired: 1 in, 5 out]
        n130 = case shown="\"QUIT\"" w179 {
          tunnel: w178 -> [_ w182]
          tunnel: [_ w180] -> w177
          frame "False", Default {
          }
          frame "QUIT" {
            n131 = Variant To Data(type=TRUE ("close FP?"), Variant=w182) -> (data=w180:bool)  [unwired: 1 in, 1 out]
            n132 = property on="QUIT" class="Bool (strict)"("Val(Sgnl)"=w180) -> ()  [unwired: 2 in, 2 out]
          }
        }
      }
      event "SCIENTIFICA Button": Value Change {
        n133 = event-data() -> ()  [unwired: 1 in, 5 out]
        n134 = call <vilib>:"Open URL in Default Browser (string).vi"("URL"="http://www.scientifica.uk.com/") -> ()  [unwired: 5 in, 2 out]
      }
      event "rotate.enable": Value Change {
        n135 = event-data() -> ()  [unwired: 1 in, 5 out]
        n136 = Select(t=T14."Enabled" ("Disabled"), s="rotate.enable", f=T14."Disabled and Grayed Out" ("Disabled")) -> (s? t:f=w187:T14)
        n137 = property on="ROTATE" class="Knob (strict)"("DisabledEnum"=w187) -> ()  [unwired: 2 in, 2 out]
      }
      event "XYZ stage settings slider tab", "advanced settings slider tab", "hist/ref slider tab", "PMT slider tab", "laser power slider tab": Mouse Enter; "XYZ stage settings slider tab", "advanced settings slider tab", "hist/ref slider tab", "PMT slider tab", "laser power slider tab": Mouse Leave {
        n138 = event-data() -> ("Type"=w193:T18, "CtlRef"=w192:refnum<vi>)  [unwired: 1 in, 1 out]
        n139 = case shown="1, Default" w194 {
          tunnel: [0 w202] -> w195
          tunnel: w193 -> [_ w201]
          tunnel: w193 -> [_ w200]
          tunnel: w192 -> [_ w199]
          tunnel: [w196 w198] -> w191
          tunnel: w190 -> [w196 _]
          frame 0 {
          }
          frame 1, Default {
            n140 = case shown="\"Mouse Leave\", Default" w201 {
              tunnel: [0 150] -> w202
              frame "Mouse Leave", Default {
              }
              frame "Mouse Enter" {
              }
            }
            n141 = Bundle("Type"=w200, "CtlRef"=w199) -> (w198:cluster{"Type":T18, "CtlRef":refnum<vi>})  [unwired: 1 in]
          }
        }
      }
      event "clear prot", "timestamp.prot", "protocol.notes": Value Change {
        n142 = event-data() -> ("CtlRef"=w209:refnum<vi>)  [unwired: 1 in, 4 out]
        n143 = property class="Ctl"(reference=w209) -> ("Label.Text"=w208:string)  [unwired: 1 in, 2 out]
        n144 = case shown="\"clear prot\"" w208 {
          tunnel: "protocol.notes" -> [w210 w212 _]
          tunnel: [w210 w211 ""] -> w206
          frame "Null", Default {
          }
          frame "timestamp.prot" {
            n145 = Get Date/Time In Seconds() -> (seconds since 1Jan1904=w215:timestamp)
            n146 = Format Date/Time String(time format string (%c)="%Y-%m-%d %H:%M:%S%2u", seconds (now)=w215) -> (date/time string=w213:string)  [unwired: 1 in]
            n147 = Concatenate Strings(w212, "\n##################\n" ("string"), w213) -> (w211:string)
          }
          frame "clear prot" {
          }
        }
        n148 = local write "protocol.notes"(w206) -> ()
      }
    }
  }
  n149 = flat-sequence {
    tunnel: w7 -> [_]
    tunnel: w5 -> [w218]
    tunnel: [w218] -> w1
    frame #0 {
      # "tab controls"
      n150 = disable-structure shown="Enabled" {
        frame Disabled {
          n151 = call "set and reset slider tabs.vi"("Set(T)/Reset(F)"=TRUE) -> ()  [unwired: 11 in]
        }
        frame Enabled {
        }
      }
      n152 = local write "scan mode main settings"(scan_mode_main_settings_tab."2D frame" ("scan mode main settings")) -> ()
      n153 = Build Array("nomin.x.pixels" ("Variable Name in")) -> (w221:string[])
      n154 = call "GFG refresh all variables.vi"("Variables to refresh"=w221) -> ()  [unwired: 11 in]
      n155 = call "init obj.vi"() -> ()  [unwired: 12 in]
      n156 = call "initialize slider tabs.vi"() -> ()  [unwired: 12 in]
      n157 = flat-sequence {
        frame #0 {
        }
        frame #1 {
          w222 = T14."Enabled" ("Disabled")
          n158 = property on="FOCUS" class="Bool (strict)"("DisabledEnum"=w222) -> ()  [unwired: 2 in, 2 out]
          n159 = property on="Record" class="Bool (strict)"("DisabledEnum"=w222) -> ()  [unwired: 2 in, 2 out]
        }
      }
    }
  }
  n160 = flat-sequence {
    tunnel: w13 -> [w225]
    tunnel: [w225] -> w10
    tunnel: w1 -> [_]
    tunnel: w10 -> [w226]
    frame #0 {
      n161 = call "close modules.vi"("close FP?"=TRUE) -> ()  [unwired: 11 in]
    }
    frame #1 {
      n162 = Not(x=w226) -> (.not. x?=w227:bool)
      n163 = call "ReadGFGandWriteToINI.vi"() -> ("error out"=w228:errorcluster)  [unwired: 11 in]
      n164 = local write "QUIT"(w227) -> ()
      n165 = call "GFG_core.vi"("error in (no error)"=w228, "Action"=enum16{"Init", "Set", "Get"}."Init") -> ()  [unwired: 11 in, 7 out]
    }
    frame #2 {
      n166 = case shown="True" TRUE {
        frame False {
          n167 = Quit LabVIEW(quit? (T)=TRUE) -> ()
        }
        frame True {
          n168 = case shown="False" FALSE {
            frame False {
            }
            frame True {
              n169 = control-ref of="This VI"() -> (w233:refnum<vi>)
              n170 = invoke class="VI" method="FP.Close"(reference=w233) -> ()  [unwired: 2 in, 3 out]
            }
          }
        }
      }
    }
  }
